vi "read_CurrentBias.vi"() -> ()   [LabVIEW 2014]
panel:
  out "Dup Aardvark Handle":i32
  out "Current":dbl
  out "error out":errorcluster
  in  "error in (no error)":errorcluster
  in  "Address (0x50)":u16=80 max=1023 format="%.0x"
  in  "Aardvark Handle":i32 min=0
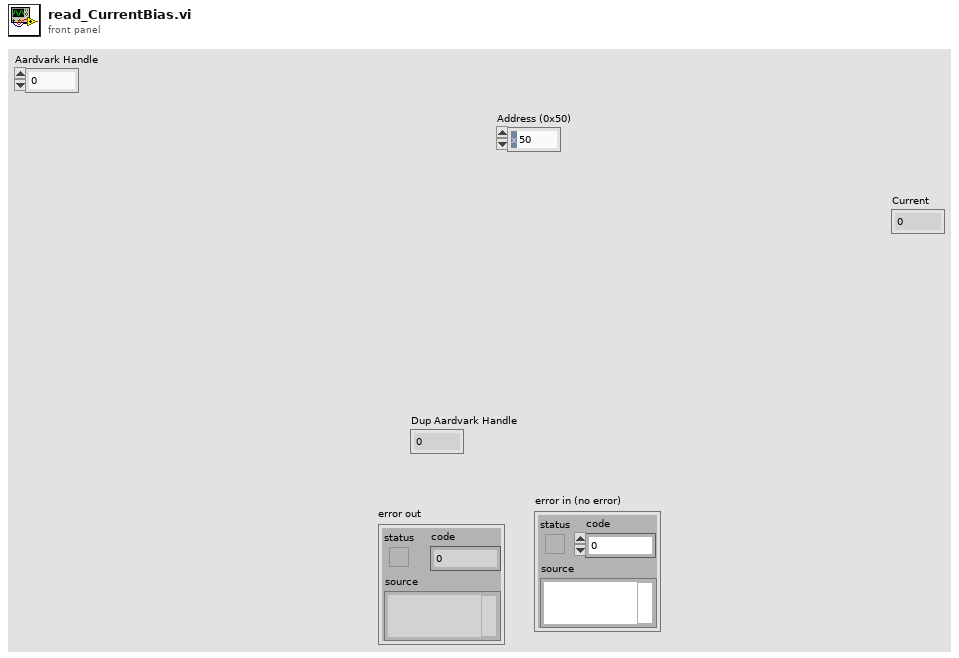
[diagram p1: front panel]
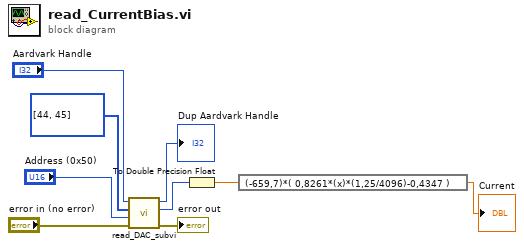
[diagram p0: block diagram]
diagram:
  n1 = call "read_DAC_subvi.vi"("error in (no error)"="error in (no error)", "Address (0x50)"="Address (0x50)", "DAC_ADD"=u8[] [44, 45], "Aardvark Handle"="Aardvark Handle") -> ("error out"=→"error out":errorcluster, "DAC Val"=w5:u16, "Dup Aardvark Handle"=→"Dup Aardvark Handle":i32)  [unwired: 3 in]
  n2 = To Double Precision Float(number=w5) -> (double precision float=w9:dbl)
  n3 = expression code="(-659,7)*( 0,8261*(x)*(1,25/4096)-0,4347 )"(w9) -> (→"Current":dbl)
